vi "Close Comm.vi"(8 "error in (no error)":errorcluster, 11 "VISA resource in":refnum<visa-resource-name>) -> (0 "error out":errorcluster)   [LabVIEW 2020, in "Global FIA milliGAT.lvlib"]
doc: "Performs an instrument error query before terminating the software connection to the instrument."
uses:
  <instrlib>/RxnRover/Global FIA milliGAT 3.14/Global FIA milliGAT.lvlib
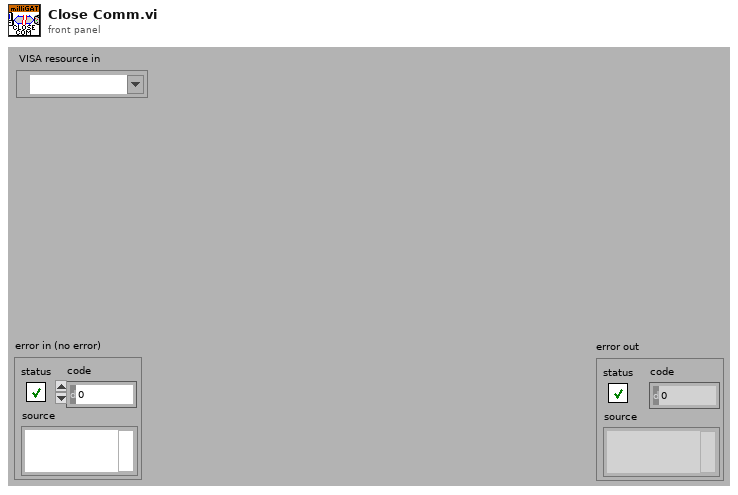
[diagram p1: front panel]
types:
  T1 = typedef "Semaphore RefNum" = refnum<k1>
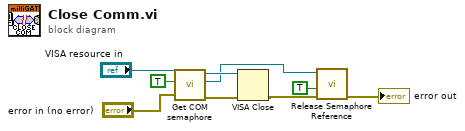
[diagram p0: block diagram]
diagram:
  n1 = call <instrlib>:"Get COM semaphore.vi"("error in (no error)"="error in (no error)", "create if not found (T)"=TRUE, "VISA resource in"="VISA resource in") -> ("error out"=w5:errorcluster, "semaphore"=w3:T1, "VISA resource out"=w6:refnum<visa-resource-name>)  [unwired: 6 in]
  n2 = VISA Close(VISA resource name=w6, error in (no error)=w5) -> (error out=w4:errorcluster)
  n3 = call <vilib>:"Release Semaphore Reference.vi"("error in (no error)"=w4, "force destroy? (F)"=TRUE, "semaphore"=w3) -> ("error out"=→"error out":errorcluster)  [unwired: 7 in, 1 out]
